vi "Open.vi"(8 "error in (no error)":errorcluster, 11 "XNET in":refnum<class "XNET_BS120x.lvclass">) -> (0 "error out":errorcluster, 3 "XNET out":refnum<class "XNET_BS120x.lvclass">)   [LabVIEW 2021, in "BS120x Driver.lvlib" / "XNET_BS120x.lvclass"]
doc: "Open an CAN bus connection to the Battery Simulator 1200 at the specified CAN Interface.\n(c) 2019 Bloomy Controls, Inc. All rights reserved."
uses:
  XNET_BS120x.lvclass
  XNET_BS120x.lvclass/XNET_BS120x.ctl
  <vilib>/xnet/xnet.llb/XNET Create Session (Frame Input Single-point).vi
  <vilib>/xnet/xnet.llb/XNET Create Session (Frame Output Single-point).vi
  <resource>/objmgr/xnet.rc
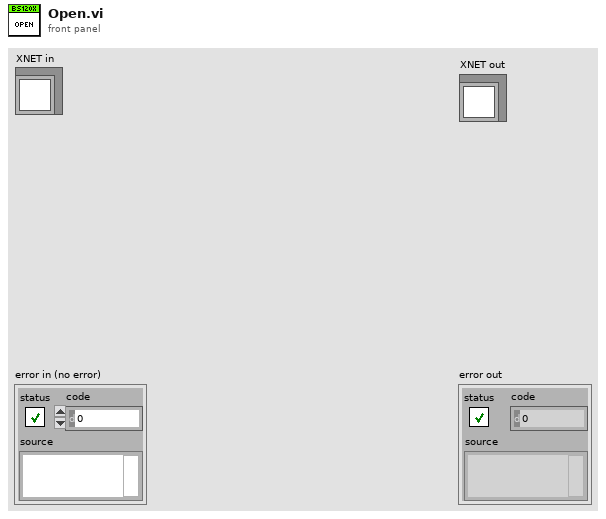
[diagram p1: front panel]
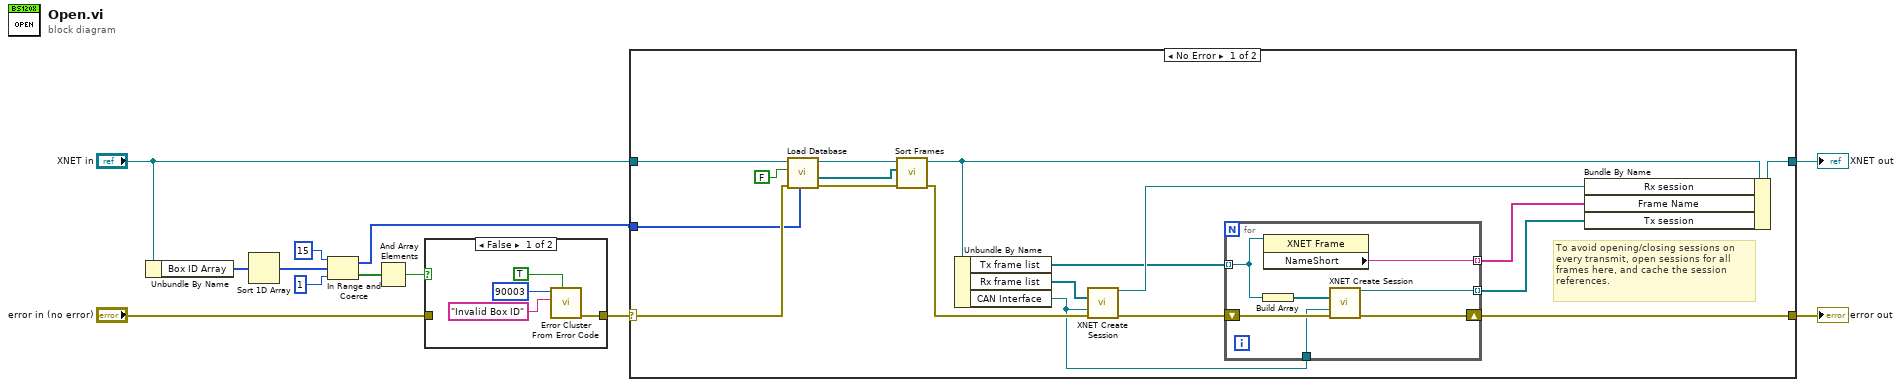
[diagram p0: block diagram]
diagram:
  n1 = Unbundle By Name("XNET in") -> ("Box ID Array"=w2:u8[])
  n2 = Sort 1D Array(array=w2) -> (sorted array=w9:u8[])
  n3 = In Range and Coerce(upper limit=u8 15, x=w9, lower limit=u8 1) -> (coerced(x)=w1:u8[], In Range?=w6:bool[])
  n4 = And Array Elements(Boolean array=w6) -> (logical AND=w5:bool)
  n5 = case shown="False" w5 {
    tunnel: "error in (no error)" -> [_ w17]
    tunnel: [w13 w17] -> w10
    frame False {
      n6 = call <vilib>:"Error Cluster From Error Code.vi"("show call chain? (False)"=TRUE, "error message (\"\")"="Invalid Box ID", "error code (0)"=90003) -> ("error out"=w13:errorcluster)  [unwired: 6 in]
    }
    frame True {
    }
  }
  n7 = case shown="No Error" w10 {
    selector: w10 -> [w29 w44]
    tunnel: [w25 w44] -> w12
    tunnel: "XNET in" -> [w20 w43]
    tunnel: [w27 w43] -> w4
    tunnel: w1 -> [w19 _]
    frame No Error {
      # "To avoid opening/closing sessions on\nevery transmit, open sessions for all\nframes here, and cache the session\nreferences."
      n8 = call-dynamic "Load Database.vi"("Box ID Array"=w19, "error in (no error)"=w29, "Calibration Mode"=FALSE, "Battery Simulator 1200 Driver in"=w20) -> ("error out"=w28:errorcluster, "Specific Frames"=w30:refnum<k21>[], "Battery Simulator 1200 Driver out"=w18:refnum<class "XNET_BS120x.lvclass">)  [unwired: 4 in, 1 out]
      n9 = call "Sort Frames.vi"("error in (no error)"=w28, "Frames"=w30, "CAN in"=w18) -> ("error out"=w33:errorcluster, "CAN out"=w32:refnum<class "XNET_BS120x.lvclass">)  [unwired: 7 in]
      n10 = Unbundle By Name(w32) -> ("Tx frame list"=w24:refnum<k21>[], "Rx frame list"=w35:refnum<k21>[], "CAN Interface"=w23:refnum<k21>)
      n11 = call-poly <vilib>:"XNET Create Session.vi"("frame list"=w35, "interface"=w23, "error in (no error)"=w33) -> ("session out"=w34:refnum<k21>, "error out"=w26:errorcluster)  [unwired: 1 in, 10 out]
      n12 = for {
        shift-right: [w41] -> w25
        shift-left: w26 -> [w42]
        tunnel: w24 -> [w38] mode=indexing
        tunnel: w23 -> [w39]
        tunnel: [w37] -> w22 mode=indexing
        tunnel: [w36] -> w21 mode=indexing
        n13 = Build Array(w38) -> (w40:refnum<k21>[])
        n14 = property class="XNET Frame"(reference=w38) -> ("NameShort"=w37:string)  [unwired: 1 in, 2 out]
        n15 = call-poly <vilib>:"XNET Create Session.vi"("frame list"=w40, "interface"=w39, "error in (no error)"=w42) -> ("session out"=w36:refnum<k21>, "error out"=w41:errorcluster)  [unwired: 1 in, 10 out]
      }
      n16 = Bundle By Name(cluster=w32, "Rx session"=w34, "Frame Name"=w22, "Tx session"=w21) -> (w27:refnum<class "XNET_BS120x.lvclass">)
    }
    frame Error {
    }
  }
  "error out" <- w12
  "XNET out" <- w4
